vi "LitePoint_VSAConfig_Waveforms.vi"(8 "error in (no error)":errorcluster, 10 "WaveformBW":u16(ring) items=["20 MHz", "100 MHz"], 11 "VISA resource name":refnum<visa-resource-name>="LitePoint_IQxstream") -> (0 "error out":errorcluster, 3 "VISA resource name out":refnum<visa-resource-name>="LitePoint_IQxstream")   [LabVIEW 2020, in "LitePoints.lvlib"]
uses:
  LitePoints.lvlib
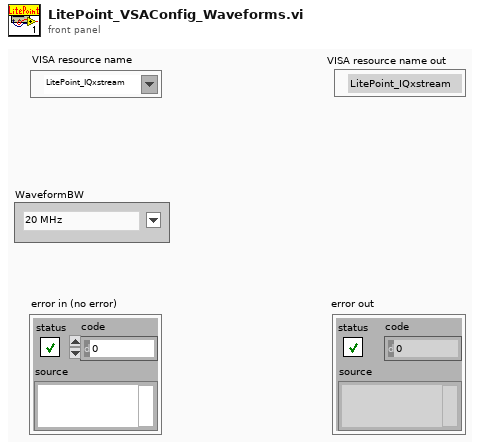
[diagram p1: front panel]
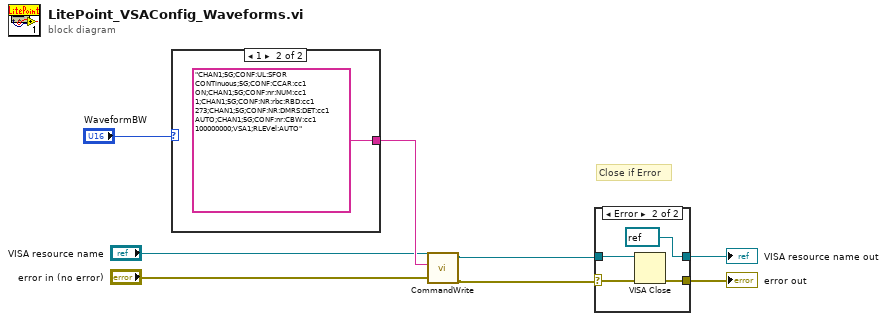
[diagram p0: block diagram]
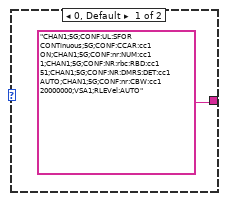
[diagram p2: hidden frame]
diagram:
  # "Close if Error"
  n1 = case shown="1" "WaveformBW" {
    tunnel: ["CHAN1;5G;CONF:UL:SFOR CONTinuous;5G;CONF:CCAR:cc1 ON;CHAN1;5G;CONF:nr:NUM:cc1 1;CHAN1;5G;CONF:NR:rbc:RBD:cc1 51;CHAN1;5G;CONF:NR:DMRS:DET:cc1 AUTO;CHAN1;5G;CONF:nr:CBW:cc1 20000000;VSA1;RLEVel:AUTO" "CHAN1;5G;CONF:UL:SFOR CONTinuous;5G;CONF:CCAR:cc1 ON;CHAN1;5G;CONF:nr:NUM:cc1 1;CHAN1;5G;CONF:NR:rbc:RBD:cc1 273;CHAN1;5G;CONF:NR:DMRS:DET:cc1 AUTO;CHAN1;5G;CONF:nr:CBW:cc1 100000000;VSA1;RLEVel:AUTO"] -> w6
    frame 0, Default {
    }
    frame 1 {
    }
  }
  n2 = call "CommandWrite.vi"("error in (no error)"="error in (no error)", "Write Buffer"=w6, "VISA resource name"="VISA resource name") -> ("error out"=w2:errorcluster, "VISA resource name out"=w3:refnum<visa-resource-name>)  [unwired: 7 in]
  n3 = case shown="Error" w2 {
    selector: w2 -> [w11 w14]
    tunnel: w3 -> [w12 w15]
    tunnel: [w12 refnum<visa-resource-name> refnum ("VISA resource name out")] -> w8
    tunnel: [w11 w13] -> w7
    frame No Error {
    }
    frame Error {
      n4 = VISA Close(VISA resource name=w15, error in (no error)=w14) -> (error out=w13:errorcluster)
    }
  }
  "VISA resource name out" <- w8
  "error out" <- w7
